vi "onConnection.vi"(8 "error in (no error)":errorcluster, 11 "LocalQueueConnection in":refnum<class "LocalQueueConnection.lvclass">) -> (0 "error out":errorcluster, 3 "LocalQueueConnection":refnum<class "LocalQueueConnection.lvclass">)   [LabVIEW 2013, in "MQTT_Queue.lvlib" / "LocalQueueConnection.lvclass"]
uses:
  LocalQueueConnection.lvclass
  MQTT_Connection/Connection/Connection.lvclass
  LocalQueueConnection.lvclass/LocalQueueConnection.ctl
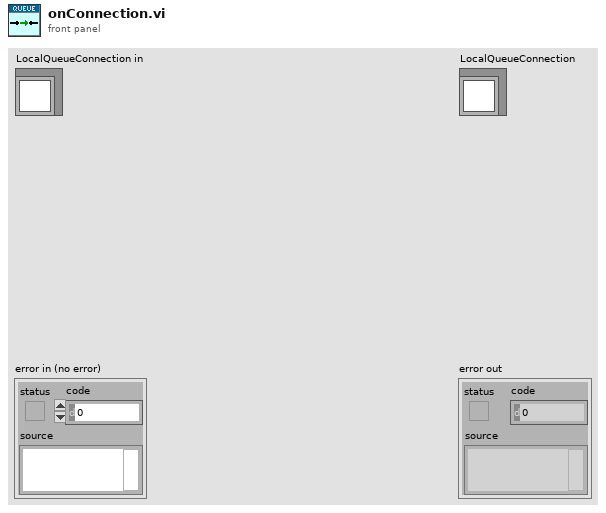
[diagram p1: front panel]
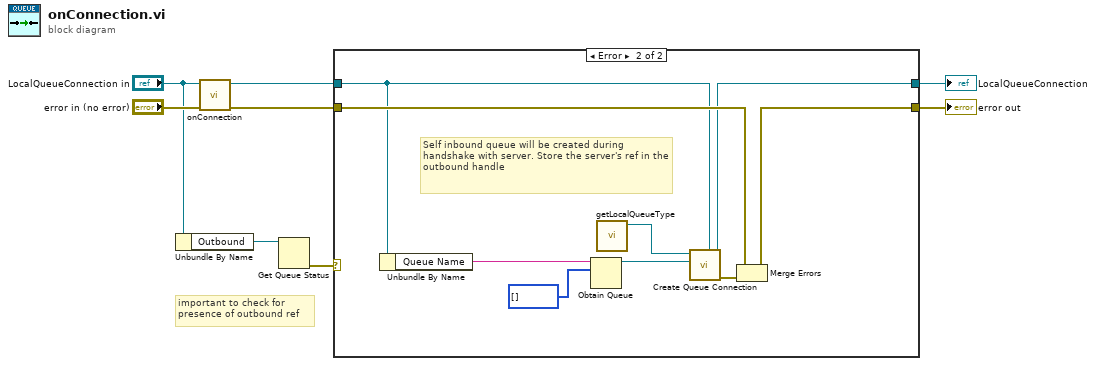
[diagram p0: block diagram]
diagram:
  # "important to check for\npresence of outbound ref"
  n1 = Unbundle By Name("LocalQueueConnection in") -> ("Outbound"=w2:refnum<queue>)
  n2 = call-parent "onConnection.vi"("error in (no error)"="error in (no error)", "Connection in"="LocalQueueConnection in") -> ("error out"=w7:errorcluster, "Connection out"=w5:refnum<class "LocalQueueConnection.lvclass">)  [unwired: 8 in]
  n3 = Get Queue Status(queue=w2) -> (error out=w1:errorcluster)  [unwired: 2 in, 7 out]
  n4 = case shown="Error" w1 {
    tunnel: w7 -> [w9 w18]
    tunnel: [w9 w17] -> w6
    tunnel: w5 -> [w10 w15]
    tunnel: [w10 w16] -> w4
    frame No Error {
    }
    frame Error {
      # "Self inbound queue will be created during handshake with server. Store the server's ref in the outbound handle"
      n5 = Unbundle By Name(w15) -> ("Queue Name"=w13:string)
      n6 = Obtain Queue(name (unnamed)=w13, element data type=u8[] [] ("Bytes Stream")) -> (queue out=w11:refnum<queue>)  [unwired: 3 in, 2 out]
      n7 = call "getLocalQueueType.vi"() -> ("Queue Type"=w12:refnum<queue>)  [unwired: 11 in]
      n8 = call "Create Queue Connection.vi"("LocalQueueConnection in"=w15, "Outbound"=w11, "Inbound"=w12) -> ("error out"=w19:errorcluster, "LocalQueueConnection"=w16:refnum<class "LocalQueueConnection.lvclass">)  [unwired: 7 in]
      n9 = Merge Errors(w18, w19) -> (w17:errorcluster)
    }
  }
  "error out" <- w6
  "LocalQueueConnection" <- w4
